vi "topat.vi"() -> ()   [LabVIEW 2015]
panel:
  in  "toplaust 2":dbl(slide)=1.0 scale=-1.0..1.0
  in  "x 4":dbl(slide)=1.0 scale=-1.0..1.0
  in  "x 3":dbl(slide)=1.0 scale=-1.0..1.0
  in  "x 2":dbl(slide)=1.0 scale=-1.0..1.0
  in  "x":dbl(slide)=1.0 scale=-1.0..1.0
  in  "toplaust":dbl(slide)=-0.8163265306122449 scale=-1.0..1.0
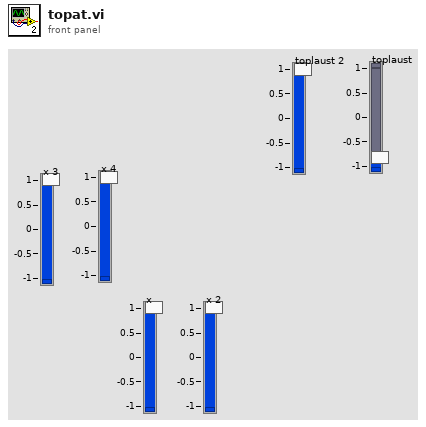
[diagram p1: front panel]
types:
  T1 = typedef "WPI_DigitalInputDevRef.ctl" = cluster{"DevStatus":errorcluster, "DIO Channel":T2}
  T2 = typedef "FPGA_DIOChannel.ctl" = enum8{"DIO 0", "DIO 1", "DIO 2", "DIO 3", "DIO 4", "DIO 5", "DIO 6", "DIO 7", "DIO 8", "DIO 9", "DIO MXP 0", "DIO MXP 1", "DIO MXP 2", "DIO MXP 3", "DIO MXP 4", "DIO MXP 5", "DIO MXP 6", "DIO MXP 7", "DIO MXP 8", "DIO MXP 9", "DIO MXP 10", "DIO MXP 11", "DIO MXP 12", "DIO MXP 13", "DIO MXP 14", "DIO MXP 15", "Invalid"}
  T3 = typedef "WPI_MotorControlDeviceRef.ctl" = cluster{"DeviceStatus":errorcluster, "Type":T4, "PWM":cluster{"PWM Channel":T5, "DeadBand":T6}, "CAN":cluster{"Device Number":u8, "Control Mode":T7, "Semaphore":T8, "Max Vout":dbl, "TalonSRX Control Mode":T9}, "Invert":bool}
  T4 = typedef "WPI_MotorControlType.ctl" = enum16{"PWM", "CAN", "CANTalonSRX"}
  T5 = typedef "FPGA_DIOPWMChannel.ctl" = enum8{"PWM 0", "PWM 1", "PWM 2", "PWM 3", "PWM 4", "PWM 5", "PWM 6", "PWM 7", "PWM 8", "PWM 9", "PWM MXP 0", "PWM MXP 1", "PWM MXP 2", "PWM MXP 3", "PWM MXP 4", "PWM MXP 5", "PWM MXP 6", "PWM MXP 7", "PWM MXP 8", "PWM MXP 9", "Invalid"}
  T6 = typedef "WPI_PWMDeadband.ctl" = cluster{"Name":string, "maxPositivePwm":i32, "minPositivePwm":i32, "centerPwm":i32, "maxNegativePwm":i32, "minNegativePwm":i32, "angularRange":u16}
  T7 = typedef "WPI_CANJaguar_ControlMode.ctl" = enum8{"Percent VBus", "Current", "Speed", "Position", "Voltage"}
  T8 = typedef "Semaphore RefNum" = refnum<k1>
  T9 = typedef "WPI_CANTalonSRX_APIControlMode.ctl" = enum8{"Percent VBus", "Speed", "Position", "Slave", "Unchanged / Invalid", "Voltage Compensation", "Current", "Motion Profile"}
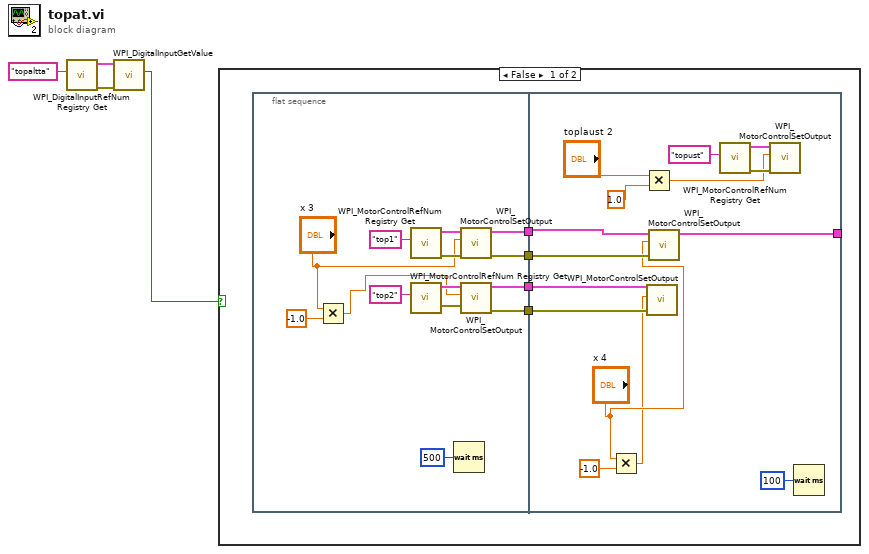
[diagram p0: block diagram]
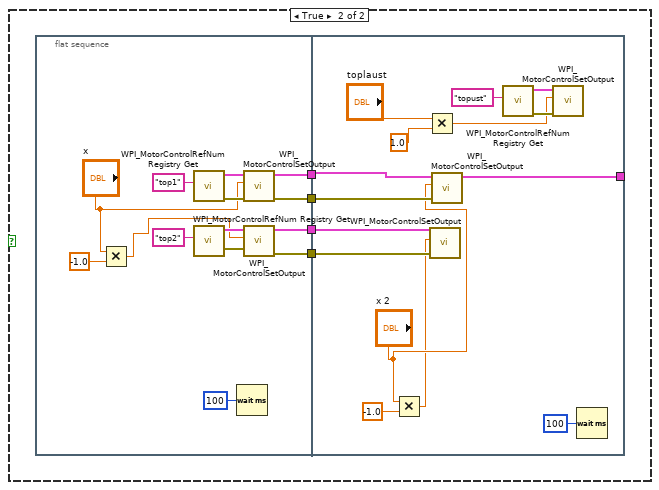
[diagram p2: hidden frame]
diagram:
  n1 = call <vilib>:"WPI_DigitalInputRefNum Registry Get.vi"("refnum name"="topaltta") -> ("error out"=w2:errorcluster, "DigitalInputDevRef"=w4:T1)  [unwired: 9 in]
  n2 = call <vilib>:"WPI_DigitalInputGetValue.vi"("error in (no error)"=w2, "DigitalInputDevRef"=w4) -> ("Value"=w1:bool)  [unwired: 7 in, 2 out]
  n3 = case shown="False" w1 {
    frame False {
      n4 = flat-sequence {
        tunnel: [w16] -> w8
        tunnel: [w15] -> w7
        tunnel: [w14] -> w6
        tunnel: [w13] -> w5
        tunnel: w8 -> [w30]
        tunnel: w7 -> [w29]
        tunnel: w6 -> [w28]
        tunnel: w5 -> [w27]
        tunnel: [w26] -> _
        frame #0 {
          n5 = Multiply(x="x 3", y=-1.0) -> (x*y=w11:dbl)
          n6 = call <vilib>:"WPI_MotorControlRefNum Registry Get.vi"("refnum name"="top1") -> ("error out"=w22:errorcluster, "MotorControlDevRef"=w21:T3)  [unwired: 9 in]
          n7 = call <vilib>:"WPI_MotorControlRefNum Registry Get.vi"("refnum name"="top2") -> ("error out"=w19:errorcluster, "MotorControlDevRef"=w18:T3)  [unwired: 9 in]
          n8 = Wait (ms)(milliseconds to wait=u32 500) -> ()  [unwired: 1 out]
          n9 = call <vilib>:"WPI_MotorControlSetOutput.vi"("error in (no error)"=w22, "Output"="x 3", "MotorControlDevRef"=w21) -> ("error out"=w13:errorcluster, "MotorControlDevRef"=w16:T3)  [unwired: 6 in, 1 out]
          n10 = call <vilib>:"WPI_MotorControlSetOutput.vi"("error in (no error)"=w19, "Output"=w11, "MotorControlDevRef"=w18) -> ("error out"=w14:errorcluster, "MotorControlDevRef"=w15:T3)  [unwired: 6 in, 1 out]
        }
        frame #1 {
          n11 = Multiply(x="x 4", y=-1.0) -> (x*y=w23:dbl)
          n12 = Multiply(x="toplaust 2", y=1.0) -> (x*y=w32:dbl)
          n13 = call <vilib>:"WPI_MotorControlSetOutput.vi"("error in (no error)"=w28, "Output"=w23, "MotorControlDevRef"=w29) -> ()  [unwired: 6 in, 3 out]
          n14 = call <vilib>:"WPI_MotorControlSetOutput.vi"("error in (no error)"=w27, "Output"="x 4", "MotorControlDevRef"=w30) -> ("MotorControlDevRef"=w26:T3)  [unwired: 6 in, 2 out]
          n15 = call <vilib>:"WPI_MotorControlRefNum Registry Get.vi"("refnum name"="topust") -> ("error out"=w37:errorcluster, "MotorControlDevRef"=w36:T3)  [unwired: 9 in]
          n16 = call <vilib>:"WPI_MotorControlSetOutput.vi"("error in (no error)"=w37, "Output"=w32, "MotorControlDevRef"=w36) -> ()  [unwired: 6 in, 3 out]
          n17 = Wait (ms)(milliseconds to wait=u32 100) -> ()  [unwired: 1 out]
        }
      }
    }
    frame True {
      n18 = flat-sequence {
        tunnel: [w49] -> w41
        tunnel: [w48] -> w40
        tunnel: [w47] -> w39
        tunnel: [w46] -> w38
        tunnel: w41 -> [w63]
        tunnel: w40 -> [w62]
        tunnel: w39 -> [w61]
        tunnel: w38 -> [w60]
        tunnel: [w59] -> _
        frame #0 {
          n19 = Multiply(x="x", y=-1.0) -> (x*y=w44:dbl)
          n20 = call <vilib>:"WPI_MotorControlRefNum Registry Get.vi"("refnum name"="top1") -> ("error out"=w55:errorcluster, "MotorControlDevRef"=w54:T3)  [unwired: 9 in]
          n21 = call <vilib>:"WPI_MotorControlRefNum Registry Get.vi"("refnum name"="top2") -> ("error out"=w52:errorcluster, "MotorControlDevRef"=w51:T3)  [unwired: 9 in]
          n22 = Wait (ms)(milliseconds to wait=u32 100) -> ()  [unwired: 1 out]
          n23 = call <vilib>:"WPI_MotorControlSetOutput.vi"("error in (no error)"=w55, "Output"="x", "MotorControlDevRef"=w54) -> ("error out"=w46:errorcluster, "MotorControlDevRef"=w49:T3)  [unwired: 6 in, 1 out]
          n24 = call <vilib>:"WPI_MotorControlSetOutput.vi"("error in (no error)"=w52, "Output"=w44, "MotorControlDevRef"=w51) -> ("error out"=w47:errorcluster, "MotorControlDevRef"=w48:T3)  [unwired: 6 in, 1 out]
        }
        frame #1 {
          n25 = Multiply(x="x 2", y=-1.0) -> (x*y=w56:dbl)
          n26 = Multiply(x="toplaust", y=1.0) -> (x*y=w65:dbl)
          n27 = call <vilib>:"WPI_MotorControlSetOutput.vi"("error in (no error)"=w61, "Output"=w56, "MotorControlDevRef"=w62) -> ()  [unwired: 6 in, 3 out]
          n28 = call <vilib>:"WPI_MotorControlSetOutput.vi"("error in (no error)"=w60, "Output"="x 2", "MotorControlDevRef"=w63) -> ("MotorControlDevRef"=w59:T3)  [unwired: 6 in, 2 out]
          n29 = call <vilib>:"WPI_MotorControlRefNum Registry Get.vi"("refnum name"="topust") -> ("error out"=w70:errorcluster, "MotorControlDevRef"=w69:T3)  [unwired: 9 in]
          n30 = call <vilib>:"WPI_MotorControlSetOutput.vi"("error in (no error)"=w70, "Output"=w65, "MotorControlDevRef"=w69) -> ()  [unwired: 6 in, 3 out]
          n31 = Wait (ms)(milliseconds to wait=u32 100) -> ()  [unwired: 1 out]
        }
      }
    }
  }
